vi "PID.vi"() -> ()   [LabVIEW 2024]
uses:
  <vilib>/addons/control/pid/pid.llb/PID Advanced (DBL).vi
  <vilib>/addons/control/pid/NI_PID_pid.lvlib
panel:
  in  "milliseconds to wait":u32=5
  out "Waveform Chart":dbl(graph)=255.0
  in  "stop":bool
  in  "output range":cluster{"output high":dbl, "output low":dbl}={"output high"=255.0, "output low"=0.0} {"output low" format="%.2f"; "output high" format="%.2f"}
  out "output":dbl=255.0 format="%.2f"
  out "dt out (s)":dbl=0.006000000284984708 format="%.3f"
  in  "dt (s)":dbl=-1.0 format="%.3f"
  in  "PID gains":T1={"proportional gain (Kc)"=-25.0, "integral time (Ti, min)"=0.1, "derivative time (Td, min)"=0.0} {"derivative time (Td, min)" format="%.3f"; "integral time (Ti, min)" format="%.3f"; "proportional gain (Kc)" format="%.3f"}
  in  "setpoint range":cluster{"setpoint high":dbl, "setpoint low":dbl}={"setpoint high"=50.0, "setpoint low"=0.0} {"setpoint high" format="%.2f"; "setpoint low" format="%.2f"}
  in  "process variable":dbl=26.7 format="%.2f"
  in  "setpoint":dbl=25.0 format="%.2f"
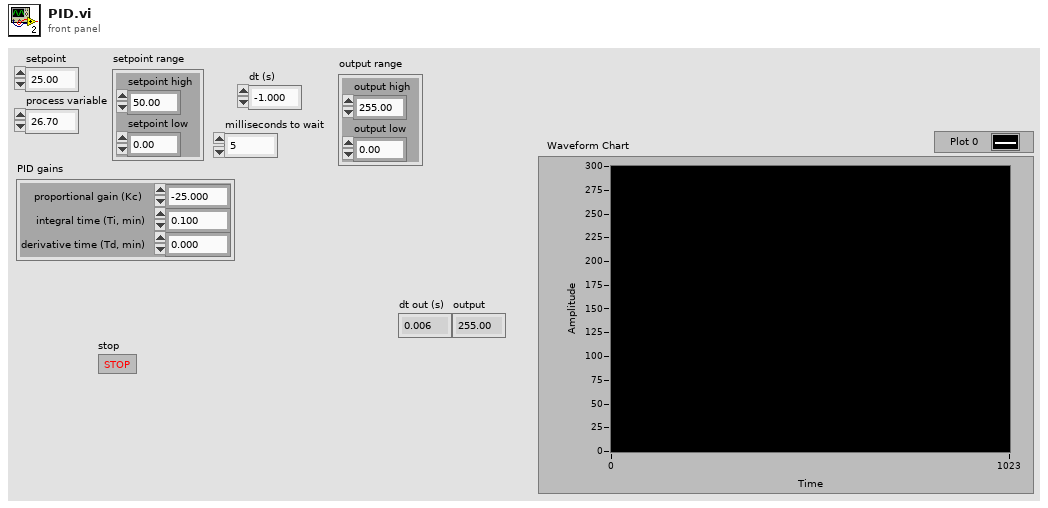
[diagram p1: front panel]
types:
  T1 = cluster{"proportional gain (Kc)":dbl, "integral time (Ti, min)":dbl, "derivative time (Td, min)":dbl}
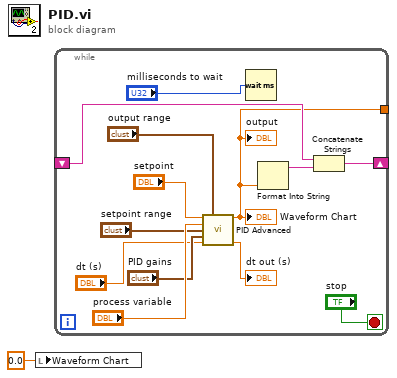
[diagram p0: block diagram]
diagram:
  n1 = local write "Waveform Chart"(0.0 ("Waveform Chart")) -> ()
  n2 = while {
    tunnel: [w9] -> _
    shift-right: [w13] -> _
    shift-left: _ -> [w11]
    stop <- "stop" stop-if-true
    n3 = call-poly <vilib>:"PID Advanced.vi"("setpoint"="setpoint", "output range"="output range", "process variable"="process variable", "setpoint range"="setpoint range", "PID gains"="PID gains", "dt (s)"="dt (s)") -> ("output"=w9:dbl, "dt out (s)"=→"dt out (s)":dbl)  [unwired: 8 in]
    "output" <- w9
    "Waveform Chart" <- w9
    n4 = Wait (ms)(milliseconds to wait="milliseconds to wait") -> ()  [unwired: 1 out]
    n5 = Format Into String(w9) -> (resulting string=w12:string)  [unwired: 3 in, 1 out]
    n6 = Concatenate Strings(w11, w12) -> (w13:string)
  }
